vi "SetLimits.vi"(8 "error in (no error)":errorcluster, 11 "KEITHLEY in":refnum<class "KEITHLEY.lvclass">) -> (0 "error out":errorcluster, 3 "KEITHLEY out":refnum<class "KEITHLEY.lvclass">)   [LabVIEW 2024, in "KEITHLEY.lvclass"]
uses:
  KEITHLEY.lvclass
  KEITHLEY.lvclass/KEITHLEY.ctl
  MainClass/PowerSupply.lvclass
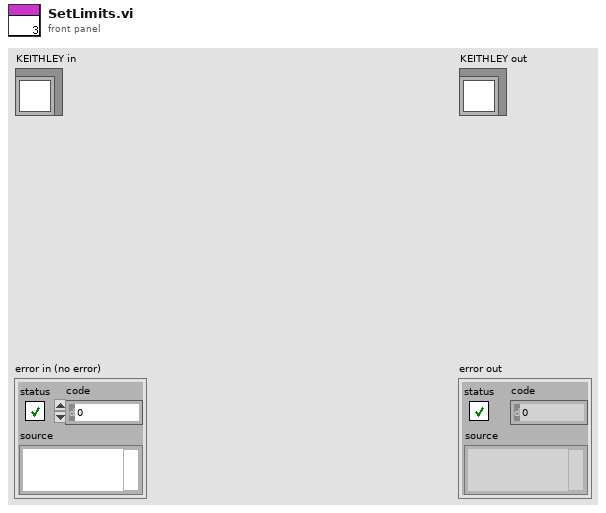
[diagram p1: front panel]
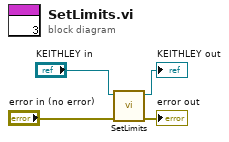
[diagram p0: block diagram]
diagram:
  n1 = call-parent "SetLimits.vi"("error in (no error)"="error in (no error)", "PowerSupply in"="KEITHLEY in") -> ("error out"=→"error out":errorcluster, "PowerSupply out"=→"KEITHLEY out":refnum<class "KEITHLEY.lvclass">)  [unwired: 8 in]
